vi "FGV.vi"(1 "Enum":T1, 6 "Param In":T3={"number of samples/ch 2"=100000, FALSE, "sound format"={"sample rate (S/s)"=22050.0, "number of channels"=2, "bits per sample"=16}}) -> (2 "Param Out":T3)   [LabVIEW 2017]
uses:
  <vilib>/sound2/lvsound2.llb/Sound Data Format.ctl
  set_get.ctl
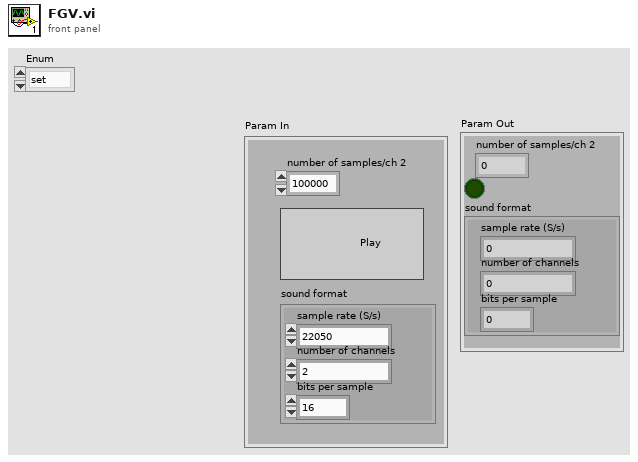
[diagram p1: front panel]
types:
  T1 = typedef "set_get.ctl" = enum16{"set", "get"}
  T2 = typedef "Sound Data Format.ctl" = cluster{"sample rate (S/s)":dbl, "number of channels":i32, "bits per sample":i32}
  T3 = cluster{"number of samples/ch 2":i32, bool, "sound format":T2}
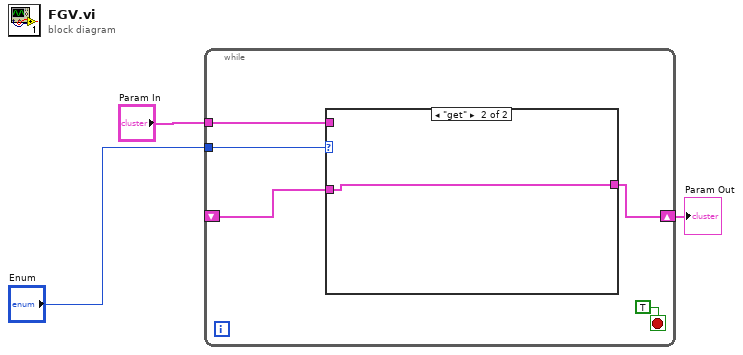
[diagram p0: block diagram]
diagram:
  n1 = while {
    tunnel: "Param In" -> [w7]
    shift-right: [w5] -> w2
    shift-left: _ -> [w6]
    tunnel: "Enum" -> [w4]
    stop <- TRUE ("stop") stop-if-true
    n2 = case shown="\"get\"" w4 {
      tunnel: w7 -> [w9 _]
      tunnel: [w9 w10] -> w5
      tunnel: w6 -> [_ w10]
      frame "set", Default {
      }
      frame "get" {
      }
    }
  }
  "Param Out" <- w2
